vi "Subvi rise edge.vi"(11 "Input":bool) -> (3 "Output":bool)   [LabVIEW 2017]
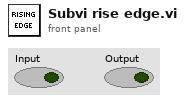
[diagram p1: front panel]
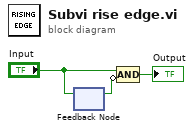
[diagram p0: block diagram]
diagram:
  n1 = feedback #1() -> (w2:bool)  [unwired: 1 in]
  n2 = feedback-in #1("Input") -> ()
  n3 = Compound Arithmetic op=AND("Input", invert w2) -> (→"Output":bool)
